vi "Unregister use event.vi"(8 "error in (no error)":errorcluster, 11 "GUI Builder in":refnum<class "GUI Builder.lvclass">) -> (0 "error out":errorcluster)   [LabVIEW 2021, in "App-Builder Library.lvlib" / "GUI Builder.lvclass"]
uses:
  GUI Builder.lvclass
  GUI Builder.lvclass/GUI Builder.ctl
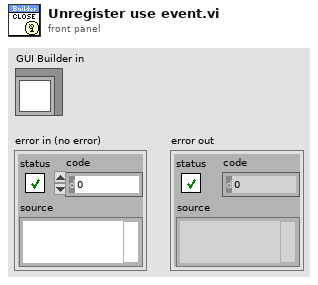
[diagram p1: front panel]
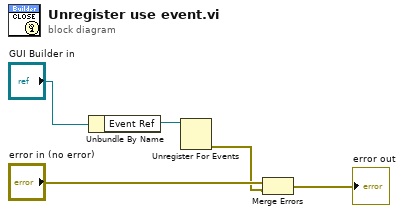
[diagram p0: block diagram]
diagram:
  n1 = Unbundle By Name("GUI Builder in") -> ("Event Ref"=w1:refnum<event-registration>)
  n2 = Unregister For Events(event registration refnum=w1) -> (error out=w3:errorcluster)  [unwired: 1 in]
  n3 = Merge Errors("error in (no error)", w3) -> (→"error out":errorcluster)
